vi "GFGevent listener template.vi"() -> ()   [LabVIEW 2012, in "GFG library.lvlib"]
doc: "SciScan 1.2 160622"
uses:
  GFG library.lvlib
  <vilib>/Utility/VariantDataType/Type.ctl
  <vilib>/Utility/VariantDataType/VariantType.lvlib
panel:
  in  "stop":bool
  out "SourceVI":string
  out "Variable Name":string
  out "Variant":variant
  out "date/time string":string
  out "Data Type":T1
  in  "error in (no error)":errorcluster
  out "error out":errorcluster
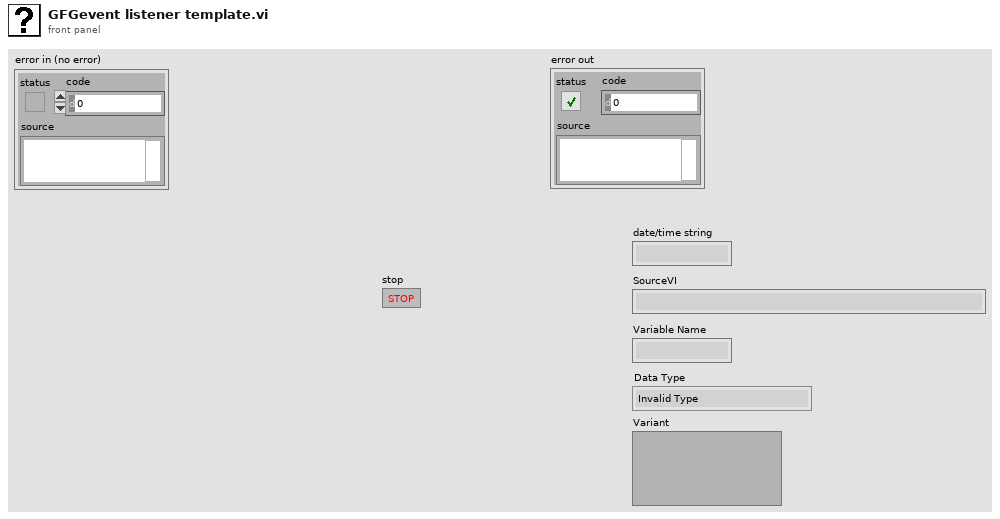
[diagram p1: front panel]
types:
  T1 = typedef "VariantType.lvlib/Type.ctl" = enum8{"Invalid Type", "Void", "I8", "I16", "I32", "I64", "U8", "U16", "U32", "U64", "Single Float", "Double Float", "Extended Float", "Single Complex", "Double Complex", "Extended Complex", "Enum U8", "Enum U16", "Enum U32", "Enum U64", "Single Float With Unit", "Double Float With Unit", "Extended Float With Unit", "Single Complex with Unit", "Double Complex with Unit", "Extended Complex with Unit", "Boolean", "String", "Path", "Picture", "Tag", "Array", "Cluster", "Variant", "LV Variant", "Waveform", "Timestamp", "Digital Waveform", "Digital Data", "ExpressData", "Refnum", "External Data", "VI", "Poly VI", "LabVIEW Class Instance", "Fixed Point"}
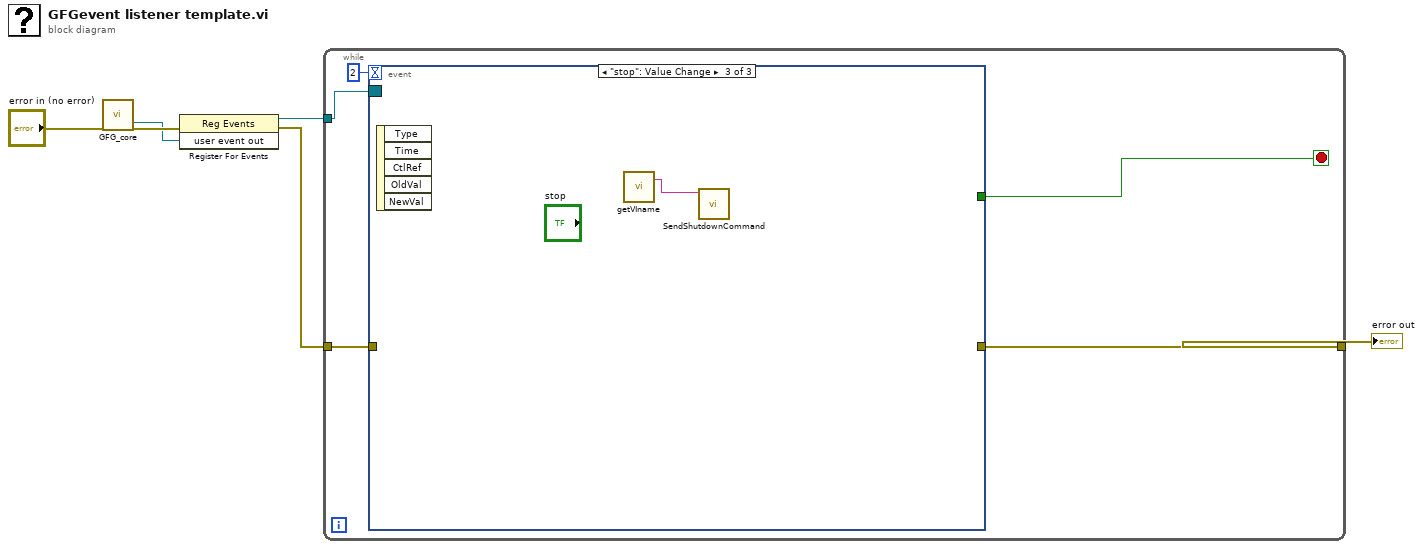
[diagram p0: block diagram]
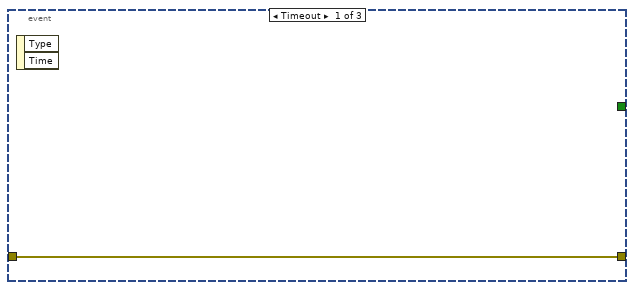
[diagram p2: hidden frame]
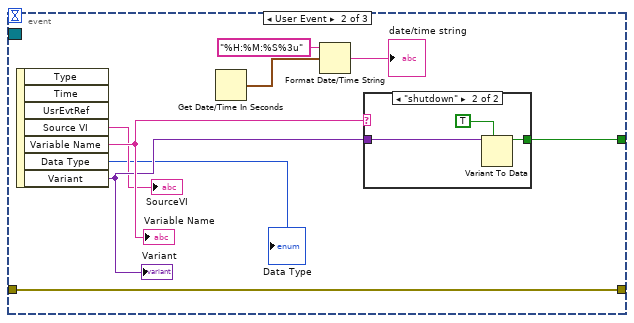
[diagram p3: hidden frame]
diagram:
  n1 = call "GFG_core.vi"("error in (no error)"="error in (no error)") -> ("user event out"=w2:refnum<user-event>, "error out"=w3:errorcluster)  [unwired: 12 in, 5 out]
  n2 = register-events(error in=w3, w2) -> (reference out=w1:refnum<event-registration>, error out=w5:errorcluster)  [unwired: 1 in]
  n3 = while {
    tunnel: w1 -> [w11]
    tunnel: w5 -> [w9]
    tunnel: [w8] -> w6
    stop <- w10 stop-if-true
    n4 = event shown="[2] \"stop\": Value Change" {
      selector: w11 -> [_ _ _]
      dyn-events: _ -> [_ _ _]
      timeout: 2 -> [_ _ _]
      tunnel: [_ w18 _] -> w10
      tunnel: w9 -> [w12 w13 _]
      tunnel: [w12 w13 _] -> w8
      event Timeout {
        n5 = event-data() -> ()  [unwired: 1 in, 2 out]
      }
      event User Event {
        n6 = event-data() -> ("Source VI"=→"SourceVI":string, "Variable Name"=w21:string, "Data Type"=→"Data Type":T1, "Variant"=w20:variant)  [unwired: 1 in, 3 out]
        "Variable Name" <- w21
        "Variant" <- w20
        n7 = Get Date/Time In Seconds() -> (seconds since 1Jan1904=w15:timestamp)
        n8 = Format Date/Time String(time format string (%c)="%H:%M:%S%3u", seconds (now)=w15) -> (date/time string=→"date/time string":string)  [unwired: 1 in]
        n9 = case shown="\"shutdown\"" w21 {
          tunnel: w20 -> [_ w24]
          tunnel: [_ w22] -> w18
          frame "False", Default {
          }
          frame "shutdown" {
            n10 = Variant To Data(type=TRUE ("want seconds? (F)"), Variant=w24) -> (data=w22:bool)  [unwired: 1 in, 1 out]
          }
        }
      }
      event "stop": Value Change {
        n11 = event-data() -> ()  [unwired: 1 in, 5 out]
        n12 = call "getVIname.vi"() -> ("VI name"=w25:string)  [unwired: 19 in]
        n13 = call "SendShutdownCommand.vi"("Source VI"=w25) -> ()  [unwired: 11 in]
      }
    }
  }
  "error out" <- w6
